vi "Register Entity.vi"(8 "error in (no error)":errorcluster, 10 "Entity":refnum<class "Entity.lvclass">, 11 "Entity Manager in":refnum<class "Entity Manager.lvclass">) -> (0 "error out":errorcluster, 3 "Entity Manager out":refnum<class "Entity Manager.lvclass">)   [LabVIEW 2020, in "Conditu2.lvlib" / "Entity Manager.lvclass"]
uses:
  Entity Manager.lvclass
  Entity/Entity.lvclass
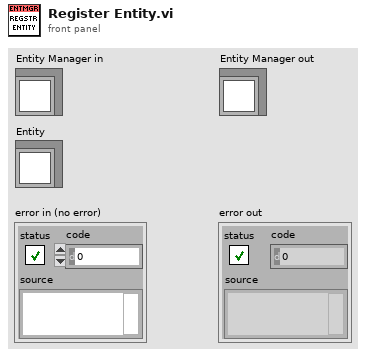
[diagram p1: front panel]
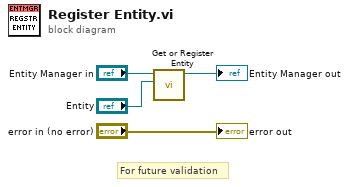
[diagram p0: block diagram]
diagram:
  # "For future validation"
  n1 = call "Get or Register Entity.vi"("Entity"="Entity", "Entity Manager in"="Entity Manager in") -> ("Entity Manager out"=→"Entity Manager out":refnum<class "Entity Manager.lvclass">)  [unwired: 7 in, 2 out]
  "error out" <- "error in (no error)"
